vi "Agilent VNA Set Sweep Type.vi"(6 "Channel":i8=1 min=1 max=99 step=1, 7 "Agilent VNA":T1, 8 "error in (no error)":errorcluster, 10 "Sweep Type":T2, 11 "VISA Resource Name":refnum<visa-resource-name>) -> (0 "error out":errorcluster, 3 "dup VISA Resource Name":refnum<visa-resource-name>)   [LabVIEW 2011]
doc: "This VI for the HP8753B is used to set the meausurement format."
uses:
  TypeDefs/Agilent VNA Sweep Type.ctl
  TypeDefs/Agilent VNA Instrument Info.ctl
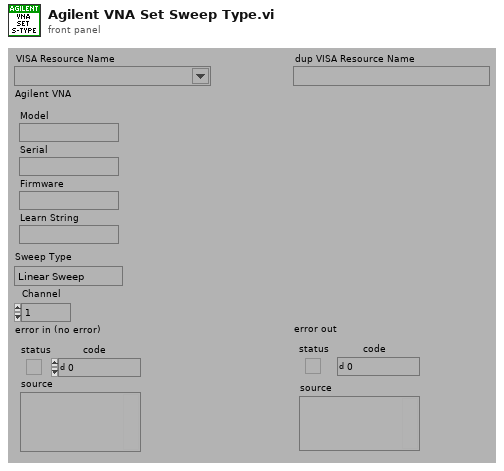
[diagram p1: front panel]
types:
  T1 = typedef "Agilent VNA Instrument Info.ctl" = cluster{"Model":string, "Serial":string, "Firmware":string, "Learn String":string}
  T2 = typedef "Agilent VNA Sweep Type.ctl" = enum32{"Linear Sweep", "Logarithmic Sweep", "Frequency List", "CW Time Sweep", "Power Sweep"}
  T3 = typedef "Agilent VNA Model.ctl" = enum16{"Not Supported", "8510X", "8719X", "8720X", "8722X", "8753X", "ENA", "PNA", "Field Fox"}
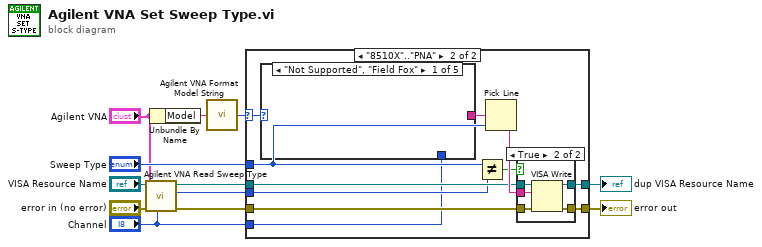
[diagram p0: block diagram]
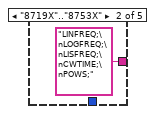
[diagram p3: hidden frame]
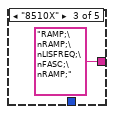
[diagram p4: hidden frame]
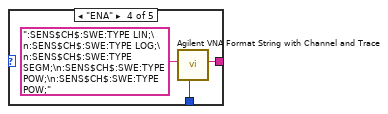
[diagram p5: hidden frame]
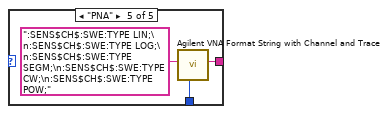
[diagram p6: hidden frame]
diagram:
  n1 = call "Agilent VNA Read Sweep Type.vi"("Channel"="Channel", "Agilent VNA"="Agilent VNA", "error in (no error)"="error in (no error)", "VISA Resource Name"="VISA Resource Name") -> ("error out"=w8:errorcluster, "Sweep Type"=w5:T2, "dup VISA Resource Name"=w7:refnum<visa-resource-name>)  [unwired: 5 out]
  n2 = Unbundle By Name("Agilent VNA") -> ("Model"=w3:string)
  n3 = call "Agilent VNA Format Model String.vi"("Model"=w3) -> ("Model"=w1:T3)
  n4 = case shown="\"8510X\"..\"PNA\"" w1 {
    selector: w1 -> [_ w15]
    tunnel: [w14 w25] -> w12
    tunnel: [w13 w24] -> w11
    tunnel: w8 -> [w13 w22]
    tunnel: w7 -> [w14 w21]
    tunnel: "Sweep Type" -> [_ w20]
    tunnel: w5 -> [_ w19]
    tunnel: "Channel" -> [_ w16]
    frame "Not Supported", "Field Fox" {
    }
    frame "8510X".."PNA" {
      n5 = case shown="\"Not Supported\", \"Field Fox\"" w15 {
        tunnel: [_ "LINFREQ;\nLOGFREQ;\nLISFREQ;\nCWTIME;\nPOWS;" "RAMP;\nRAMP;\nLISFREQ;\nFASC;\nRAMP;" w29 w32] -> w17
        tunnel: w16 -> [_ _ _ w28 w31]
        frame "Not Supported", "Field Fox" {
        }
        frame "8719X".."8753X" {
        }
        frame "8510X" {
        }
        frame "ENA" {
          n6 = call "Agilent VNA Format String with Channel and Trace.vi"("Channel"=w28, "String"=":SENS$CH$:SWE:TYPE LIN;\n:SENS$CH$:SWE:TYPE LOG;\n:SENS$CH$:SWE:TYPE SEGM;\n:SENS$CH$:SWE:TYPE POW;\n:SENS$CH$:SWE:TYPE POW;") -> ("String Out"=w29:string)  [unwired: 1 in, 6 out]
        }
        frame "PNA" {
          n7 = call "Agilent VNA Format String with Channel and Trace.vi"("Channel"=w31, "String"=":SENS$CH$:SWE:TYPE LIN;\n:SENS$CH$:SWE:TYPE LOG;\n:SENS$CH$:SWE:TYPE SEGM;\n:SENS$CH$:SWE:TYPE CW;\n:SENS$CH$:SWE:TYPE POW;") -> ("String Out"=w32:string)  [unwired: 1 in, 6 out]
        }
      }
      n8 = Not Equal?(x=w20, y=w19) -> (x != y?=w18:bool)
      n9 = Pick Line(multi-line string=w17, line index=w20) -> (output string=w23:string)  [unwired: 1 out]
      n10 = case shown="True" w18 {
        tunnel: [w35 w40] -> w25
        tunnel: [w34 w39] -> w24
        tunnel: w23 -> [_ w38]
        tunnel: w22 -> [w34 w37]
        tunnel: w21 -> [w35 w36]
        frame False {
        }
        frame True {
          n11 = VISA Write(VISA resource name=w36, write buffer=w38, error in (no error)=w37) -> (VISA resource name out=w40:refnum<visa-resource-name>, error out=w39:errorcluster)  [unwired: 1 out]
        }
      }
    }
  }
  "dup VISA Resource Name" <- w12
  "error out" <- w11
